vi "DAQNavi Create Channel(CI-Count Value).vi"(0 "task in":i32=-1, 5 "physical channels":string="DemoDevice,BID#0/cntr0", 11 "error in (no error)":errorcluster) -> (4 "task out":i32, 15 "error out":errorcluster)   [LabVIEW 2020]
uses:
  DAQNavi_LV.dll
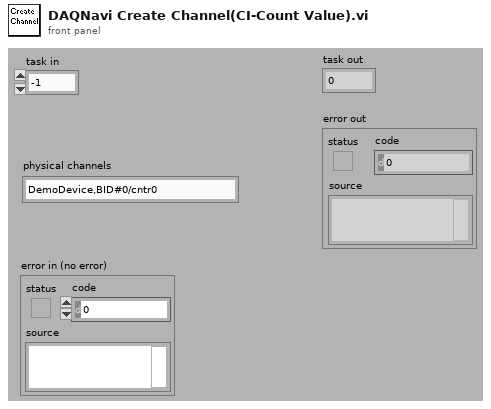
[diagram p1: front panel]
types:
  T1 = enum16{"InstantAI", "OneBufferedAI", "StreamingAI", "StaticAO", "OneWaveformAO", "StreamingAO", "InstantDI", "DIInterrupt", "StaticDO", "EventCounter", "FreqMeter", "OneShot", "TimerPulse", "PwMeter", "PwModulator", "WaveformAI"}
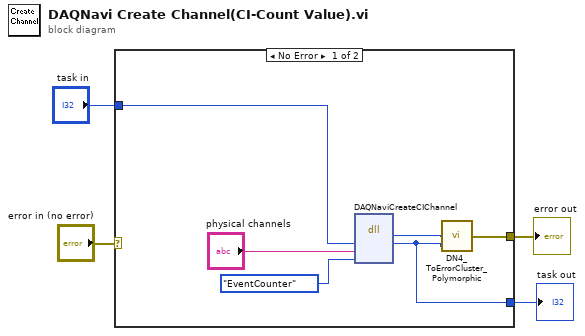
[diagram p0: block diagram]
diagram:
  n1 = case shown="No Error" "error in (no error)" {
    selector: "error in (no error)" -> [_ w11]
    tunnel: "task in" -> [w10 w12]
    tunnel: [w7 w11] -> w2
    tunnel: [w5 w12] -> w1
    frame No Error {
      n2 = dll-call lib="DAQNavi_LV.dll" fn="DAQNaviCreateCIChannel"("taskID"=w10, "physicalChannel"="physical channels", "TaskType"=T1."EventCounter") -> ("return type"=w8:i32, "taskID"=w5:i32)  [unwired: 4 in, 3 out]
      n3 = call "DN4_ToErrorCluster_Polymorphic.vi"("task id"=w5, "error code"=w8) -> ("error out"=w7:errorcluster)  [unwired: 3 out]
    }
    frame Error {
    }
  }
  "error out" <- w2
  "task out" <- w1
